vi "fpgaAcquire.vi"(1 "Command FIFO":refnum<k21>, 2 "Circular Buffer Mem":refnum<k21>, 3 "circular buffer length":u32=300, 5 "FPGA I/O In":refnum<k21>="IO Module\\AI A0", 6 "Timing FIFO":refnum<k21>, 7 "channel on/off":bool, 9 "Trigger":i16=1500, 11 "Samples to Acquire":u32=95, 12 "Is Test Pulse?":bool, 13 "# of pretrigger":u32=15, 14 "timing":u64) -> ()   [LabVIEW 2012]
uses:
  <vilib>/rvi/eio/common/nirviEmuTemplateMethod_errors.vi
  <vilib>/rvi/DataTransferAndStorage/Container/Common/niFpgaContainerExecOnDevCompGetState.vi
  <vilib>/rvi/Emulation/niFpgaSctlEmulationGetInTimedLoop.vi
  <vilib>/rvi/DataTransferAndStorage/Container/Common/niFpgaContainerGetUniqueNameForEmu.vi
  <vilib>/rvi/FIFO/Fifo_Resource/nirvififoEmulationSetSize.vi
  <vilib>/rvi/errors/niFpgaSetErrorForExecOnDevCompSimple.vi
  <vilib>/rvi/eio/common/nirviEmuReportErrorAndStop.vi
  <vilib>/rvi/Emulation/niFpgaSctlEmulationFifoFullMgr.vi
  <vilib>/rvi/Emulation/niFpgaSctlEmulationResourceMgr.vi
  <vilib>/rvi/interface/RandomDataEmulation/nirviRandomDataFPGAFIFO.vi
  <vilib>/rvi/interface/RandomDataEmulation/niFpgaRandomDataHandleErrors.vi
  <vilib>/eio/EIONode/EIONode.xnode
  <vilib>/rvi/DataTransferAndStorage/Container/XNode/niFpgaContainer.xnode
  <vilib>/rvi/FIFO/Fifo_Resource/niFpgaFifoEmulationRefIn.vi
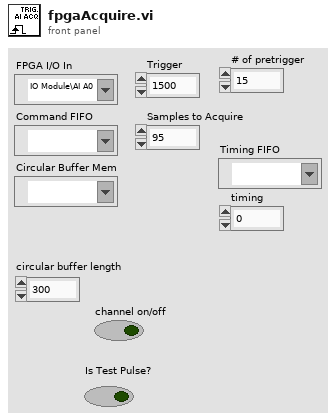
[diagram p1: front panel]
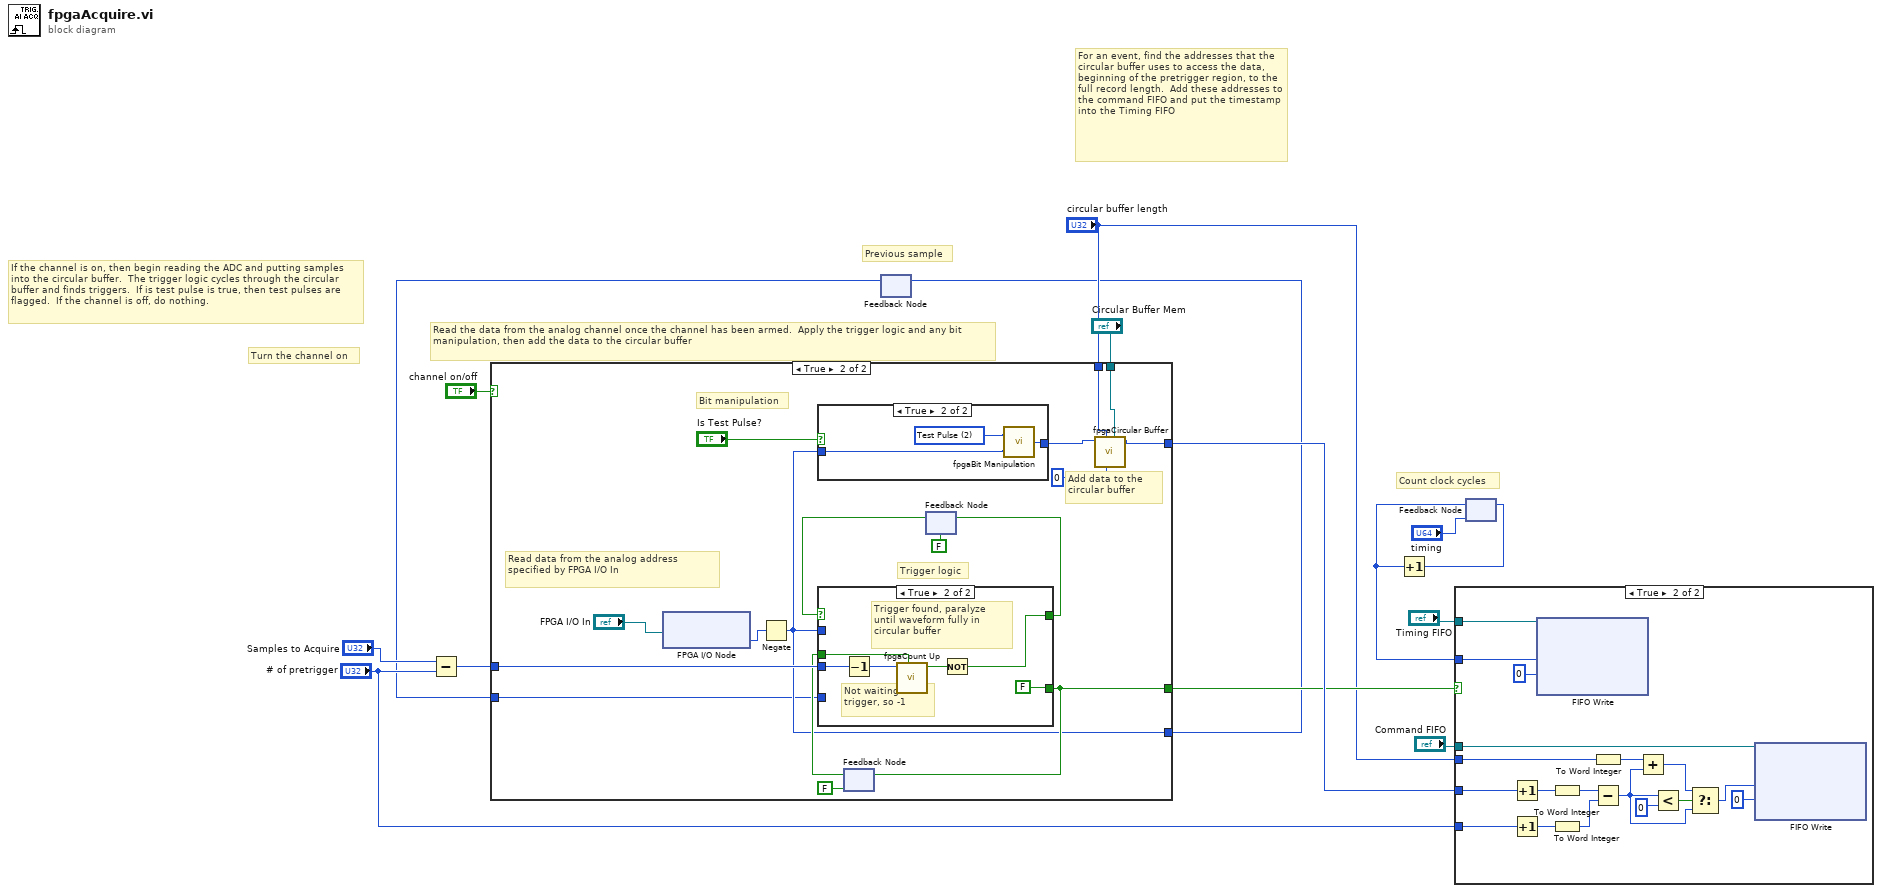
[diagram p0: block diagram]
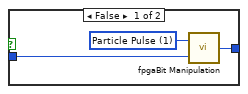
[diagram p4: hidden frame]
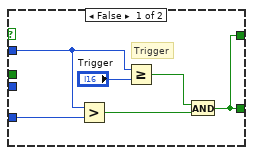
[diagram p5: hidden frame]
diagram:
  # "Previous sample"
  # "Count clock cycles"
  # "For an event, find the addresses that the circular buffer uses to access the data, beginning of the pretrigger region, to the full record length.  Add these addresses to the command FIFO and put the timestamp into the Timing FIFO"
  # "Read the data from the analog channel once the channel has been armed.  Apply the trigger logic and any bit manipulation, then add the data to the circular buffer"
  # "If the channel is on, then begin reading the ADC and putting samples into the circular buffer.  The trigger logic cycles through the circular buffer and finds triggers.  If is test pulse is true, then test pulses are flagged.  If the channel is off, do nothing."
  # "Turn the channel on"
  n1 = Subtract(x="Samples to Acquire", y="# of pretrigger") -> (x-y=w1:u32)
  n2 = feedback #1() -> (w2:i16)  [unwired: 1 in]
  n3 = case shown="True" "channel on/off" {
    tunnel: "Circular Buffer Mem" -> [_ w18]
    tunnel: "circular buffer length" -> [_ w19]
    tunnel: [_ w17] -> w15
    tunnel: w1 -> [_ w30]
    tunnel: [_ w25] -> w14
    tunnel: [_ w24] -> w3
    tunnel: w2 -> [_ w23]
    frame False {
    }
    frame True {
      # "Trigger logic"
      # "Read data from the analog address specified by FPGA I/O In"
      # "Add data to the circular buffer"
      # "Bit manipulation"
      n4 = xnode "FPGA I/O Node"("FPGA I/O In"="FPGA I/O In") -> ("I/O Item"=w21:i16)  [unwired: 1 out]
      n5 = Negate(x=w21) -> (-x=w24:i16)
      n6 = case shown="True" "Is Test Pulse?" {
        tunnel: w24 -> [w34 w37]
        tunnel: [w33 w36] -> w20
        frame False {
          w35 = u16 1 items=["Header Information", "Particle Pulse", "Test Pulse"] ("Pulse Type")
          n7 = call "fpgaBit Manipulation.vi"("Pulse Type"=w35, "Integer to be written"=w34) -> ("Integer Written"=w33:i16)  [unwired: 2 in]
        }
        frame True {
          w38 = u16 2 items=["Header Information", "Particle Pulse", "Test Pulse"] ("Pulse Type")
          n8 = call "fpgaBit Manipulation.vi"("Pulse Type"=w38, "Integer to be written"=w37) -> ("Integer Written"=w36:i16)  [unwired: 2 in]
        }
      }
      n9 = feedback #2(FALSE) -> (w27:bool)
      n10 = feedback #3(FALSE) -> (w29:bool)
      n11 = case shown="True" w29 {
        tunnel: w24 -> [w41 _]
        tunnel: w30 -> [_ w46]
        tunnel: w27 -> [_ w50]
        tunnel: [w43 w48] -> w28
        tunnel: [w43 FALSE] -> w25
        tunnel: w23 -> [w39 _]
        frame False {
          # "Trigger"
          n12 = Greater?(x=w41, y=w39) -> (0:w40:bool)
          n13 = Greater Or Equal?(x=w41, y="Trigger") -> (x >= y?=w42:bool)
          n14 = And(x=w42, y=w40) -> (x .and. y?=w43:bool)
        }
        frame True {
          # "Not waiting for trigger, so -1"
          # "Trigger found, paralyze until waveform fully in circular buffer"
          n15 = Decrement(x=w46) -> (x-1=w45:u32)
          n16 = call "fpgaCount Up.vi"("Reset?"=w50, "goal"=w45) -> ("Count Met"=w49:bool)  [unwired: 8 in, 1 out]
          n17 = Not(x=w49) -> (.not. x?=w48:bool)
        }
      }
      n18 = feedback-in #2(w25) -> ()
      n19 = feedback-in #3(w28) -> ()
      n20 = call "fpgaCircular Buffer.vi"("Refnum in"=w18, "Starting Address"=u32 0, "circular buffer length"=w19, "Data"=w20) -> ("Address"=w17:u32)  [unwired: 7 in]
    }
  }
  n21 = feedback-in #1(w3) -> ()
  n22 = feedback #4("timing") -> (w4:u64)
  n23 = Increment(x=w4) -> (x+1=w5:u64)
  n24 = case shown="True" w14 {
    tunnel: "Command FIFO" -> [_ w68]
    tunnel: "Timing FIFO" -> [_ w67]
    tunnel: w15 -> [_ w56]
    tunnel: "circular buffer length" -> [_ w54]
    tunnel: "# of pretrigger" -> [_ w51]
    tunnel: w4 -> [_ w53]
    frame False {
    }
    frame True {
      n25 = Increment(x=w56) -> (x+1=w62:u32)
      n26 = Increment(x=w51) -> (x+1=w52:u32)
      n27 = xnode ("FIFO Write")("Element"=w53, "Timeout"=0, "FIFO In"=w67) -> ()  [unwired: 2 out]
      n28 = To Word Integer(number=w62) -> (16bit integer=w63:i16)
      n29 = To Word Integer(number=w52) -> (16bit integer=w64:i16)
      n30 = To Word Integer(number=w54) -> (16bit integer=w61:i16)
      n31 = Subtract(x=w63, y=w64) -> (x-y=w60:i16)
      n32 = Add(x=w61, y=w60) -> (x+y=w59:i16)
      n33 = Less?(x=w60, y=i16 0) -> (x < y?=w57:bool)
      n34 = Select(t=w59, s=w57, f=w60) -> (s? t:f=w55:i16)
      n35 = xnode ("FIFO Write")("Element"=w55, "Timeout"=0, "FIFO In"=w68) -> ()  [unwired: 2 out]
    }
  }
  n36 = feedback-in #4(w5) -> ()
